vi "Analog_Output_4.vi"() -> ()   [LabVIEW 2019]
uses:
  <vilib>/DAQmx/write.llb/DAQmx Write (Analog Wfm 1Chan NSamp).vi
  <vilib>/DAQmx/create/channels.llb/DAQmx Create Channel (AO-Voltage-Basic).vi
  <vilib>/DAQmx/miscellaneous.llb/DAQmx Fill In Error Info.vi
  <vilib>/measure/NI_MABase.lvlib
panel:
  in  "physical channels":tag caption="물리적 채널"
  out "웨이브폼 그래프":waveform(dbl)(graph)
  in  "amplitude":dbl=1.0 caption="진폭" format="%0.2p"
  in  "frequency":dbl=10.0 caption="주파수" format="%0.2p"
  in  "정지버튼":bool
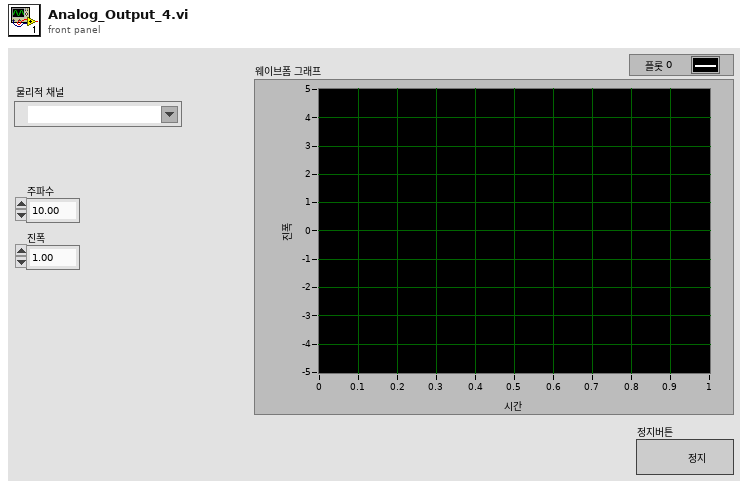
[diagram p1: front panel]
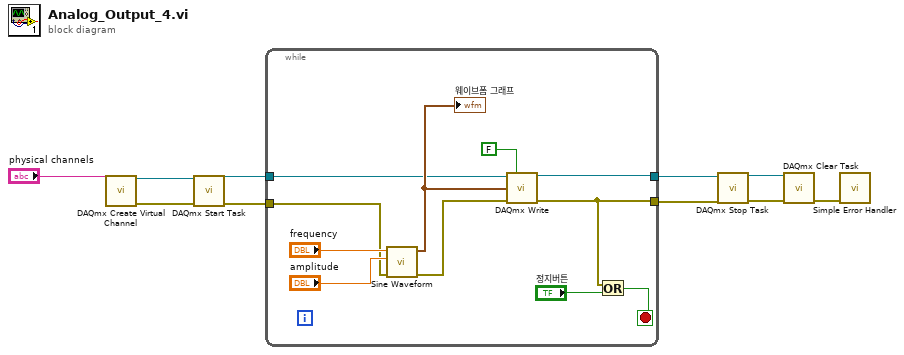
[diagram p0: block diagram]
diagram:
  n1 = call-poly <vilib>:"DAQmx Create Virtual Channel.vi"("physical channels"="physical channels") -> ("task out"=w2:refnum<k21>, "error out"=w1:errorcluster)  [unwired: 13 in]
  n2 = call <vilib>:"DAQmx Start Task.vi"("task/channels in"=w2, "error in"=w1) -> ("task out"=w10:refnum<k21>, "error out"=w9:errorcluster)  [unwired: 12 in]
  n3 = while {
    tunnel: w10 -> [w13]
    tunnel: w9 -> [w12]
    tunnel: [w18] -> w8
    tunnel: [w17] -> w7
    stop <- w21 stop-if-true
    n4 = call <vilib>:"Sine Waveform.vi"("error in (no error)"=w12, "amplitude"="amplitude", "frequency"="frequency") -> ("error out"=w11:errorcluster, "signal out"=w14:waveform(dbl))  [unwired: 7 in]
    "웨이브폼 그래프" <- w14
    n5 = call-poly <vilib>:"DAQmx Write.vi"("task/channels in"=w13, "auto start"=FALSE, "data"=w14, "error in"=w11) -> ("task out"=w18:refnum<k21>, "error out"=w17:errorcluster)  [unwired: 9 in, 1 out]
    n6 = Or(x=w17, y="정지버튼") -> (x .or. y?=w21:bool)
  }
  n7 = call <vilib>:"DAQmx Stop Task.vi"("task/channels in"=w8, "error in"=w7) -> ("task out"=w6:refnum<k21>, "error out"=w5:errorcluster)  [unwired: 12 in]
  n8 = call <vilib>:"DAQmx Clear Task.vi"("task in"=w6, "error in"=w5) -> ("error out"=w4:errorcluster)  [unwired: 13 in]
  n9 = call <vilib>:"Simple Error Handler.vi"("error in (no error)"=w4) -> ()  [unwired: 4 in, 5 out]
